vi "controlTargetPosition.vi"(7 "Set":bool, 8 "error in":errorcluster, 9 "Target Position in":dbl, 10 "axis in":u8, 11 "connection ID":refnum<k5>) -> (0 "error out":errorcluster, 1 "Target Position out":dbl, 2 "axis out":u8, 3 "connection ID":refnum<k5>)   [LabVIEW 2019]
panel:
  in  "Set Command":string="com.attocube.amc.move.setControlTargetPosition"
  in  "Get Command":string="com.attocube.amc.move.getControlTargetPosition"
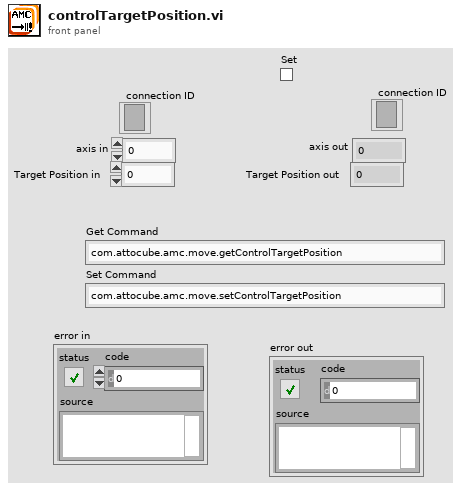
[diagram p1: front panel]
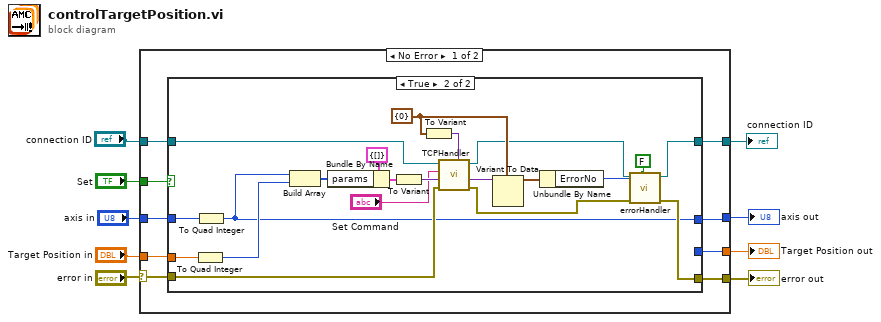
[diagram p0: block diagram]
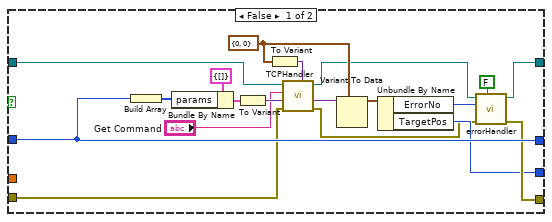
[diagram p2: hidden frame]
diagram:
  n1 = case shown="No Error" "error in" {
    selector: "error in" -> [w10 w62]
    tunnel: "axis in" -> [w15 w60]
    tunnel: [w11 w62] -> w8
    tunnel: [w13 w60] -> w7
    tunnel: "Target Position in" -> [w18 w61]
    tunnel: [w12 w61] -> w5
    tunnel: "Set" -> [w16 _]
    tunnel: [w14 w59] -> w3
    tunnel: "connection ID" -> [w17 w59]
    frame No Error {
      n2 = case shown="True" w16 {
        tunnel: [w22 w43] -> w14
        tunnel: w17 -> [w27 w53]
        tunnel: w15 -> [w29 w51]
        tunnel: [w29 w38] -> w13
        tunnel: [w28 w48] -> w11
        tunnel: [w24 _] -> w12
        tunnel: w18 -> [_ w45]
        tunnel: w10 -> [w20 w41]
        frame False {
          w25 = cluster{"ErrorNo":i16, "TargetPos":i64} {"ErrorNo"=0, "TargetPos"=0} ("input cluster")
          n3 = Build Array(w29) -> (w33:u8[])
          n4 = Bundle By Name(cluster=cluster{"params":i16[]} {"params"=[]} ("input cluster"), "params"=w33) -> (w34:cluster{"params":i16[]})
          n5 = To Variant(anything=w34) -> (Variant=w35:variant)
          n6 = To Variant(anything=w25) -> (Variant=w26:variant)
          n7 = call <userlib>:"TCPHandler.vi"("result Types"=w26, "error in (no error)"=w20, "params"=w35, "method"="Get Command", "connection ID"=w27) -> ("error out"=w19:errorcluster, "result"=w31:variant, "connection ID"=w23:refnum<k5>)  [unwired: 3 in, 1 out]
          n8 = Variant To Data(type=w25, Variant=w31) -> (data=w36:cluster{"ErrorNo":i16, "TargetPos":i64})  [unwired: 1 in, 1 out]
          n9 = Unbundle By Name(w36) -> ("ErrorNo"=w37:i16, "TargetPos"=w24:i64)
          n10 = call <userlib>:"errorHandler.vi"("show popup"=FALSE, "error in"=w19, "error number"=w37, "connection ID"=w23) -> ("error out"=w28:errorcluster, "connection ID"=w22:refnum<k5>)  [unwired: 6 in]
        }
        frame True {
          w46 = cluster{"ErrorNo":i16} {"ErrorNo"=0} ("input cluster")
          n11 = To Quad Integer(1:w45) -> (0:w39:i64)
          n12 = To Quad Integer(1:w51) -> (0:w38:i64)
          n13 = Build Array(w38, w39) -> (w55:i64[])
          n14 = Bundle By Name(cluster=cluster{"params":i64[]} {"params"=[]} ("input cluster"), "params"=w55) -> (w54:cluster{"params":i64[]})
          n15 = To Variant(anything=w54) -> (Variant=w52:variant)
          n16 = To Variant(anything=w46) -> (Variant=w47:variant)
          n17 = call <userlib>:"TCPHandler.vi"("result Types"=w47, "error in (no error)"=w41, "params"=w52, "method"="Set Command", "connection ID"=w53) -> ("error out"=w40:errorcluster, "result"=w57:variant, "connection ID"=w44:refnum<k5>)  [unwired: 3 in, 1 out]
          n18 = Variant To Data(type=w46, Variant=w57) -> (data=w50:cluster{"ErrorNo":i16})  [unwired: 1 in, 1 out]
          n19 = Unbundle By Name(w50) -> ("ErrorNo"=w49:i16)
          n20 = call <userlib>:"errorHandler.vi"("show popup"=FALSE, "error in"=w40, "error number"=w49, "connection ID"=w44) -> ("error out"=w48:errorcluster, "connection ID"=w43:refnum<k5>)  [unwired: 6 in]
        }
      }
    }
    frame Error {
    }
  }
  "error out" <- w8
  "axis out" <- w7
  "Target Position out" <- w5
  "connection ID" <- w3
